vi "Autonomous Independent.vi"() -> ()   [LabVIEW 2015]
doc: "This VI is called when autonomous begins, and will automatically be terminated when autonomous ends. You can carry out timed or sensor driven robot movement independently without needing to return to the caller."
uses:
  <vilib>/Rock Robotics/WPI/Utilities/WPI_GetSetVariantRefNum.vi
  <vilib>/Rock Robotics/Network Tables/NT Write Numeric Array.vi
  <vilib>/Rock Robotics/Network Tables/NT Read Boolean.vi
  <vilib>/Rock Robotics/Network Tables/NT Write Boolean.vi
  <vilib>/Rock Robotics/Network Tables/NT Write Number.vi
  <vilib>/Rock Robotics/Network Tables/NT Read String.vi
  <vilib>/Rock Robotics/WPI/RobotDrive/WPI_RobotDriveArcadeDrive_Standard(NoSaturation).vi
panel:
  out "Current Movement, for debugging":T1 {"Y Joystick Value" scale=1.0..-1.0; "X Joystick Value" scale=-1.0..1.0}
  in  "Array of robot movements":T2(array[cluster])=[{"X Joystick Value"=0.39393939393939403, "Y Joystick Value"=0.0, "Delay (sec)"=1.0, "Movement Name"="turn"}, {"X Joystick Value"=-0.3737373737373737, "Y Joystick Value"=0.0, "Delay (sec)"=1.0, "Movement Name"="turn back"}] {"Y Joystick Value" scale=1.0..-1.0; "X Joystick Value" scale=-1.0..1.0}
  out "Low Switch":bool
  out "High Switch":bool
  out "POT Sensor Meter":dbl(knob) scale=78.0..98.0
  out "POT Sensor Value":dbl
  # "Be sure to right-click and choose Data Operations>>Make Current Value default if you want to save the array values with the VI"
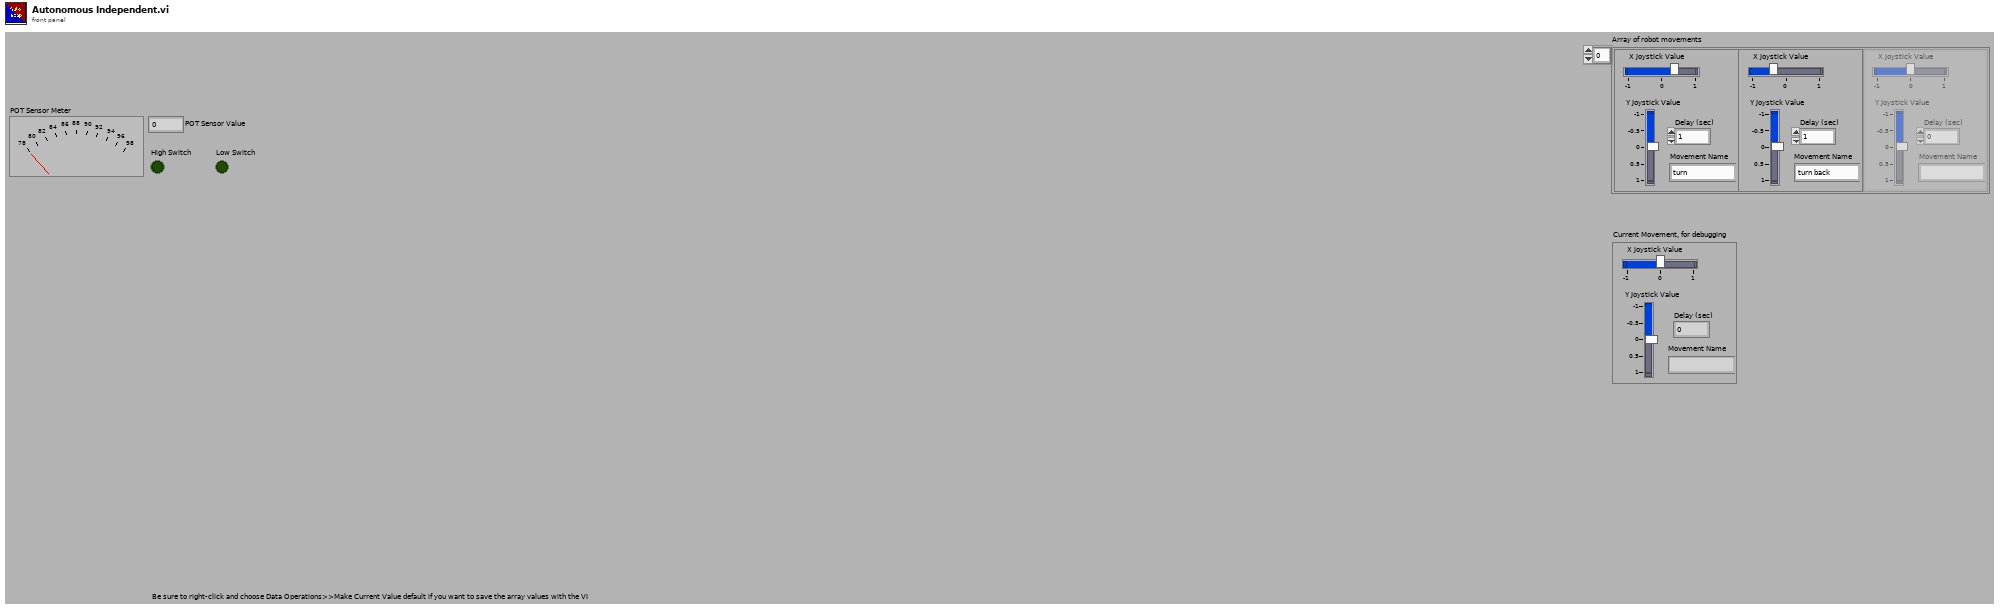
[diagram p1: front panel]
types:
  T1 = cluster{"X Joystick Value":dbl, "Y Joystick Value":dbl, "Delay (sec)":dbl, "Movement Name":string}
  T2 = cluster{"X Joystick Value":dbl, "Y Joystick Value":dbl, "Delay (sec)":dbl, "Movement Name":string}[]
  T3 = typedef "WPI_JoystickDevRef.ctl" = cluster{"Device":T4}
  T4 = typedef "WPI_JoystickDeviceEnum.ctl" = enum16{"USB 0", "USB 1", "USB 2", "USB 3", "USB 4", "USB 5"}
  T5 = typedef "WPI_SwitchDevRef.ctl" = cluster{"DevStatus":errorcluster, "DIO Channel":T6, "CntIndex":T7, "Normally Closed":bool}
  T6 = typedef "FPGA_DIOChannel.ctl" = enum8{"DIO 0", "DIO 1", "DIO 2", "DIO 3", "DIO 4", "DIO 5", "DIO 6", "DIO 7", "DIO 8", "DIO 9", "DIO MXP 0", "DIO MXP 1", "DIO MXP 2", "DIO MXP 3", "DIO MXP 4", "DIO MXP 5", "DIO MXP 6", "DIO MXP 7", "DIO MXP 8", "DIO MXP 9", "DIO MXP 10", "DIO MXP 11", "DIO MXP 12", "DIO MXP 13", "DIO MXP 14", "DIO MXP 15", "Invalid"}
  T7 = typedef "FPGA_CounterCtrSystemIndex.ctl" = enum8{"Ctr 0", "Ctr 1", "Ctr 2", "Ctr 3", "Ctr 4", "Ctr 5", "Ctr 6", "Ctr 7", "Invalid"}
  T8 = typedef "WPI_PotentiometerDevRef.ctl" = cluster{"DevStatus":errorcluster, "Analog Channel":T9, "Invert Output":bool}
  T9 = typedef "FPGA_AIChannel.ctl" = enum8{"AI 0", "AI 1", "AI 2", "AI 3", "AI MXP 0", "AI MXP 1", "AI MXP 2", "AI MXP 3", "Invalid"}
  T10 = typedef "WPI_MotorControlDeviceRef.ctl" = cluster{"DeviceStatus":errorcluster, "Type":T11, "PWM":cluster{"PWM Channel":T12, "DeadBand":T13}, "CAN":cluster{"Device Number":u8, "Control Mode":T14, "Semaphore":T15, "Max Vout":dbl, "TalonSRX Control Mode":T16}, "Invert":bool}
  T11 = typedef "WPI_MotorControlType.ctl" = enum16{"PWM", "CAN", "CANTalonSRX"}
  T12 = typedef "FPGA_DIOPWMChannel.ctl" = enum8{"PWM 0", "PWM 1", "PWM 2", "PWM 3", "PWM 4", "PWM 5", "PWM 6", "PWM 7", "PWM 8", "PWM 9", "PWM MXP 0", "PWM MXP 1", "PWM MXP 2", "PWM MXP 3", "PWM MXP 4", "PWM MXP 5", "PWM MXP 6", "PWM MXP 7", "PWM MXP 8", "PWM MXP 9", "Invalid"}
  T13 = typedef "WPI_PWMDeadband.ctl" = cluster{"Name":string, "maxPositivePwm":i32, "minPositivePwm":i32, "centerPwm":i32, "maxNegativePwm":i32, "minNegativePwm":i32, "angularRange":u16}
  T14 = typedef "WPI_CANJaguar_ControlMode.ctl" = enum8{"Percent VBus", "Current", "Speed", "Position", "Voltage"}
  T15 = typedef "Semaphore RefNum" = refnum<k1>
  T16 = typedef "WPI_CANTalonSRX_APIControlMode.ctl" = enum8{"Percent VBus", "Speed", "Position", "Slave", "Unchanged / Invalid", "Voltage Compensation", "Current", "Motion Profile"}
  T17 = typedef "WPI_RobotDriveDevRef.ctl" = cluster{"DevStatus":errorcluster, "Motors[]":T10[], "Square Inputs":bool, "Max Output":dbl}
  T18 = typedef "WPI_CounterDevRef.ctl" = cluster{"DevStatus":errorcluster, "CntIndex":T7}
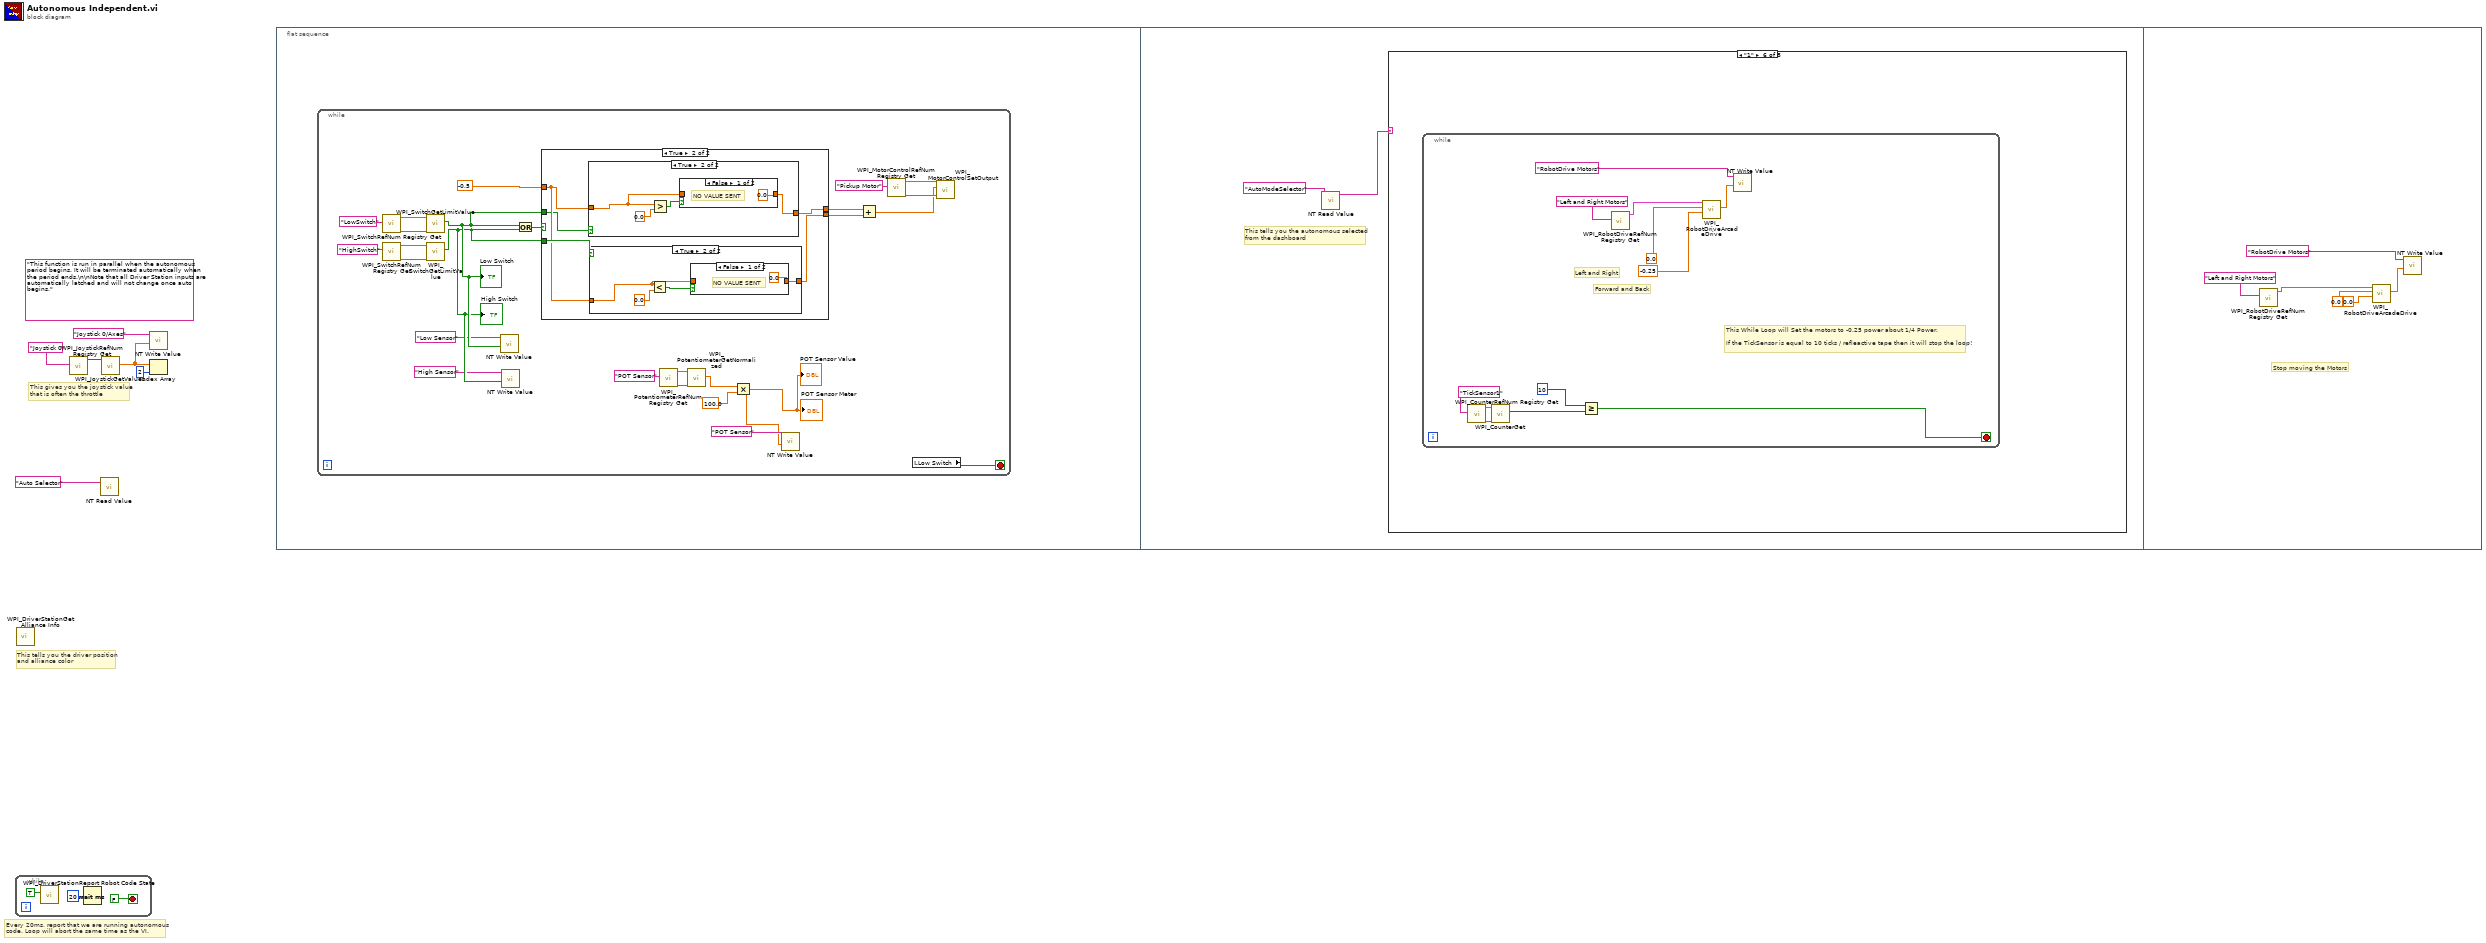
[diagram p0: block diagram]
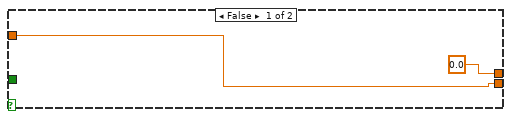
[diagram p2: hidden frame]
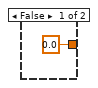
[diagram p3: hidden frame]
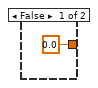
[diagram p5: hidden frame]
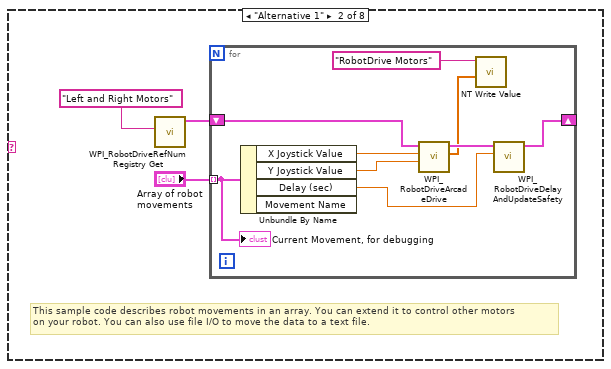
[diagram p8: hidden frame]
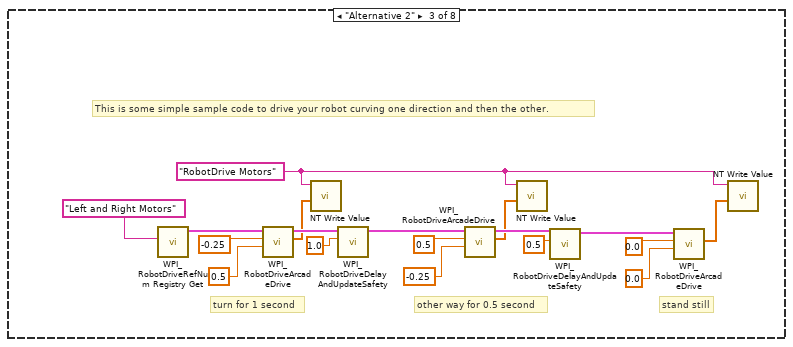
[diagram p9: hidden frame]
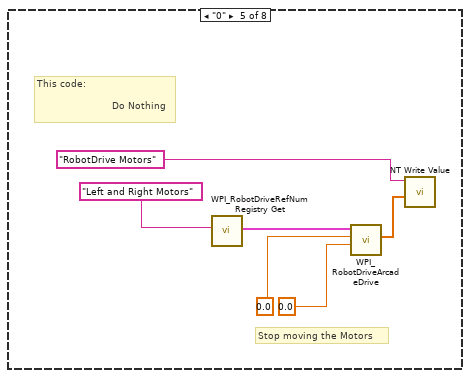
[diagram p11: hidden frame]
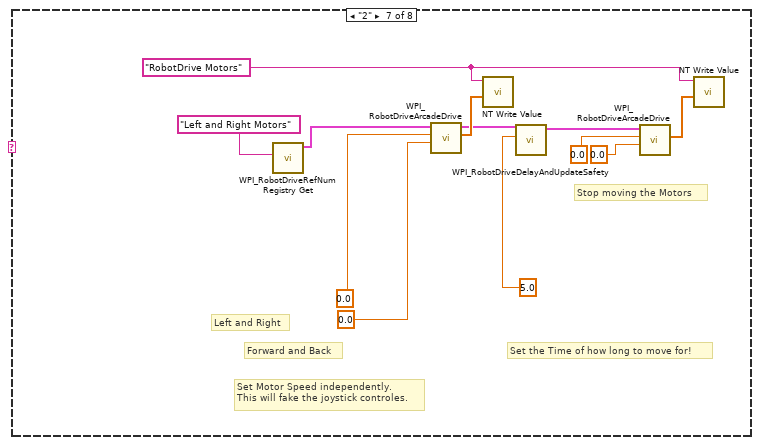
[diagram p12: hidden frame]
diagram:
  (unwired) "This function is run in parallel when the autonomous period begins. It will be terminated automatically when the period ends.\n\nNote that all Driver Station inputs are automatically latched and will not change once auto begins."
  # "Every 20ms, report that we are running autonomous\ncode. Loop will abort the same time as the VI."
  # "This gives you the joystick value\nthat is often the throttle"
  # "This tells you the driver position\nand alliance color"
  n1 = while {
    stop <- FALSE stop-if-true
    n2 = call <vilib>:"WPI_DriverStationReport Robot Code State.vi"("Autonomous"=TRUE) -> ()  [unwired: 10 in, 1 out]
    n3 = Wait (ms)(milliseconds to wait=u32 20) -> ()  [unwired: 1 out]
  }
  n4 = call <vilib>:"WPI_DriverStationGet Alliance Info.vi"() -> ()  [unwired: 12 out]
  n5 = call <vilib>:"WPI_JoystickRefNum Registry Get.vi"("refnum name"="Joystick 0") -> ("JoystickDevRef"=w5:T3)  [unwired: 1 in, 9 out]
  n6 = call-poly <vilib>:"NT Read Value.vi"("Name"="Auto Selector") -> ()  [unwired: 9 in, 2 out]
  n7 = call <vilib>:"WPI_JoystickGetValues.vi"("JoystickDevRef"=w5) -> ("Axes"=w3:dbl[])  [unwired: 6 in, 4 out]
  n8 = call-poly <vilib>:"NT Write Value.vi"("Numeric Array"=w3, "Name"="Joystick 0/Axes") -> ()  [unwired: 9 in, 1 out]
  n9 = Index Array(array=w3, index=2) -> ()  [unwired: 1 out]
  n10 = flat-sequence {
    frame #0 {
      n11 = while {
        stop <- w10 stop-if-true
        n12 = call <vilib>:"WPI_SwitchRefNum Registry Get.vi"("refnum name"="LowSwitch") -> ("error out"=w33:errorcluster, "SwitchDevRef"=w34:T5)  [unwired: 9 in]
        n13 = call <vilib>:"WPI_SwitchRefNum Registry Get.vi"("refnum name"="HighSwitch") -> ("error out"=w30:errorcluster, "SwitchDevRef"=w31:T5)  [unwired: 9 in]
        n14 = call <vilib>:"WPI_SwitchGetLimitValue.vi"("error in (no error)"=w33, "SwitchDevRef"=w34) -> ("Switch Pressed"=w18:bool)  [unwired: 7 in, 2 out]
        "Low Switch" <- w18
        n15 = call <vilib>:"WPI_SwitchGetLimitValue.vi"("error in (no error)"=w30, "SwitchDevRef"=w31) -> ("Switch Pressed"=w17:bool)  [unwired: 7 in, 2 out]
        "High Switch" <- w17
        n16 = call-poly <vilib>:"NT Write Value.vi"("Boolean"=w18, "Name"="Low Sensor") -> ()  [unwired: 9 in, 1 out]
        n17 = call-poly <vilib>:"NT Write Value.vi"("Boolean"=w17, "Name"="High Sensor") -> ()  [unwired: 9 in, 1 out]
        n18 = Or(x=w18, y=w17) -> (x .or. y?=w35:bool)
        n19 = case shown="True" w35 {
          tunnel: w18 -> [_ w40]
          tunnel: w17 -> [_ w42]
          tunnel: -0.5 ("Axes[1]") -> [w36 w41]
          tunnel: [0.0 ("Axes[1]") w39] -> w24
          tunnel: [w36 w38] -> w23
          frame False {
          }
          frame True {
            n20 = case shown="True" w40 {
              tunnel: w41 -> [_ w52]
              tunnel: [0.0 ("Axes[1]") w51] -> w39
              frame False {
              }
              frame True {
                n21 = Greater?(x=w52, y=0.0) -> (0:w53:bool)
                n22 = case shown="False" w53 {
                  tunnel: [0.0 ("Axes[1]") w56] -> w51
                  tunnel: w52 -> [_ w56]
                  frame False {
                    # "NO VALUE SENT"
                  }
                  frame True {
                  }
                }
              }
            }
            n23 = case shown="True" w42 {
              tunnel: w41 -> [_ w44]
              tunnel: [0.0 ("Axes[1]") w45] -> w38
              frame False {
              }
              frame True {
                n24 = Less?(x=w44, y=0.0) -> (x < y?=w46:bool)
                n25 = case shown="False" w46 {
                  tunnel: [0.0 ("Axes[1]") w49] -> w45
                  tunnel: w44 -> [_ w49]
                  frame False {
                    # "NO VALUE SENT"
                  }
                  frame True {
                  }
                }
              }
            }
          }
        }
        n26 = call <vilib>:"WPI_PotentiometerRefNum Registry Get.vi"("refnum name"="POT Sensor") -> ("error out"=w22:errorcluster, "PotDevRef"=w21:T8)  [unwired: 9 in]
        n27 = call <vilib>:"WPI_PotentiometerGetNormalized.vi"("error in"=w22, "PotDevRef"=w21) -> ("Normalized Value"=w14:dbl)  [unwired: 7 in, 2 out]
        n28 = Multiply(x=w14, y=100.0) -> (x*y=w12:dbl)
        "POT Sensor Value" <- w12
        "POT Sensor Meter" <- w12
        n29 = call-poly <vilib>:"NT Write Value.vi"("Numeric"=w12, "Name"="POT Sensor") -> ()  [unwired: 9 in, 1 out]
        n30 = Add(x=w24, y=w23) -> (x+y=w25:dbl)
        n31 = call <vilib>:"WPI_MotorControlRefNum Registry Get.vi"("refnum name"="Pickup Motor") -> ("error out"=w28:errorcluster, "MotorControlDevRef"=w27:T10)  [unwired: 9 in]
        n32 = local read "Low Switch"() -> (w10:bool)
        n33 = call <vilib>:"WPI_MotorControlSetOutput.vi"("error in (no error)"=w28, "Output"=w25, "MotorControlDevRef"=w27) -> ()  [unwired: 6 in, 3 out]
      }
    }
    frame #1 {
      # "This tells you the autonomous selected\nfrom the dashboard"
      n34 = call-poly <vilib>:"NT Read Value.vi"("Name"="AutoModeSelector") -> ("String"=w57:string)  [unwired: 9 in, 1 out]
      n35 = case shown="\"1\"" w57 {
        frame Default {
          # "You can put your main auto here, or you can right-click on the case and make any\nother frame be the default case."
          # "This is the frame that will execute if no selection is made, or if it is not recognized"
        }
        frame "Alternative 1" {
          # "This sample code describes robot movements in an array. You can extend it to control other motors\non your robot. You can also use file I/O to move the data to a text file."
          n36 = call <vilib>:"WPI_RobotDriveRefNum Registry Get.vi"("refnum name"="Left and Right Motors") -> ("RobotDriveDevRef"=w60:T17)  [unwired: 1 in, 9 out]
          n37 = for {
            shift-right: [w68] -> _
            shift-left: w60 -> [w69]
            tunnel: "Array of robot movements" -> [w64] mode=indexing
            n38 = Unbundle By Name(w64) -> ("X Joystick Value"=w67:dbl, "Y Joystick Value"=w66:dbl, "Delay (sec)"=w65:dbl)  [unwired: 1 out]
            n39 = call-poly <vilib>:"WPI_RobotDriveArcadeDrive.vi"("Y axis value"=w66, "X axis value"=w67, "RobotDriveDevRef"=w69) -> ("Motor Values"=w62:dbl[], "RobotDriveDevRef"=w70:T17)  [unwired: 1 in, 6 out]
            n40 = call-poly <vilib>:"NT Write Value.vi"("Numeric Array"=w62, "Name"="RobotDrive Motors") -> ()  [unwired: 9 in, 1 out]
            n41 = call <vilib>:"WPI_RobotDriveDelayAndUpdateSafety.vi"("Delay (s)"=w65, "RobotDriveDevRef"=w70) -> ("RobotDriveDevRef 2"=w68:T17)  [unwired: 8 in, 1 out]
            "Current Movement, for debugging" <- w64
          }
        }
        frame "Alternative 2" {
          w72 = "RobotDrive Motors" ("Name")
          # "This is some simple sample code to drive your robot curving one direction and then the other."
          # "stand still"
          # "other way for 0.5 second"
          # "turn for 1 second"
          n42 = call <vilib>:"WPI_RobotDriveRefNum Registry Get.vi"("refnum name"="Left and Right Motors") -> ("RobotDriveDevRef"=w88:T17)  [unwired: 1 in, 9 out]
          n43 = call-poly <vilib>:"WPI_RobotDriveArcadeDrive.vi"("Y axis value"=0.5 ("X axis value"), "X axis value"=-0.25, "RobotDriveDevRef"=w88) -> ("Motor Values"=w71:dbl[], "RobotDriveDevRef"=w81:T17)  [unwired: 1 in, 6 out]
          n44 = call-poly <vilib>:"NT Write Value.vi"("Numeric Array"=w71, "Name"=w72) -> ()  [unwired: 9 in, 1 out]
          n45 = call <vilib>:"WPI_RobotDriveDelayAndUpdateSafety.vi"("Delay (s)"=1.0, "RobotDriveDevRef"=w81) -> ("RobotDriveDevRef 2"=w82:T17)  [unwired: 8 in, 1 out]
          n46 = call-poly <vilib>:"WPI_RobotDriveArcadeDrive.vi"("Y axis value"=-0.25 ("X axis value"), "X axis value"=0.5, "RobotDriveDevRef"=w82) -> ("Motor Values"=w73:dbl[], "RobotDriveDevRef"=w83:T17)  [unwired: 1 in, 6 out]
          n47 = call-poly <vilib>:"NT Write Value.vi"("Numeric Array"=w73, "Name"=w72) -> ()  [unwired: 9 in, 1 out]
          n48 = call <vilib>:"WPI_RobotDriveDelayAndUpdateSafety.vi"("Delay (s)"=0.5, "RobotDriveDevRef"=w83) -> ("RobotDriveDevRef 2"=w84:T17)  [unwired: 8 in, 1 out]
          n49 = call-poly <vilib>:"WPI_RobotDriveArcadeDrive.vi"("Y axis value"=0.0 ("X axis value"), "X axis value"=0.0, "RobotDriveDevRef"=w84) -> ("Motor Values"=w74:dbl[])  [unwired: 1 in, 7 out]
          n50 = call-poly <vilib>:"NT Write Value.vi"("Numeric Array"=w74, "Name"=w72) -> ()  [unwired: 9 in, 1 out]
        }
        frame "Your Turn" {
        }
        frame "0" {
          # "Stop moving the Motors"
          # "This code:\n                   \n                         Do Nothing"
          n51 = call <vilib>:"WPI_RobotDriveRefNum Registry Get.vi"("refnum name"="Left and Right Motors") -> ("RobotDriveDevRef"=w89:T17)  [unwired: 1 in, 9 out]
          n52 = call-poly <vilib>:"WPI_RobotDriveArcadeDrive.vi"("Y axis value"=0.0 ("X axis value"), "X axis value"=0.0, "RobotDriveDevRef"=w89) -> ("Motor Values"=w93:dbl[])  [unwired: 1 in, 7 out]
          n53 = call-poly <vilib>:"NT Write Value.vi"("Numeric Array"=w93, "Name"="RobotDrive Motors") -> ()  [unwired: 9 in, 1 out]
        }
        frame "1" {
          n54 = while {
            stop <- w101 stop-if-true
            # "This While Loop will Set the motors to -0.25 power about 1/4 Power.\n\nIf the TickSensor is equal to 10 ticks / refleactive tape then it will stop the loop!"
            # "Forward and Back"
            # "Left and Right"
            n55 = call <vilib>:"WPI_CounterRefNum Registry Get.vi"("refnum name"="TickSensor1") -> ("error out"=w105:errorcluster, "CounterDevRef"=w104:T18)  [unwired: 9 in]
            n56 = call <vilib>:"WPI_CounterGet.vi"("error in (no error)"=w105, "CounterDevRef in"=w104) -> ("Value"=w103:i32)  [unwired: 4 in, 5 out]
            n57 = Greater Or Equal?(x=10, y=w103) -> (x >= y?=w101:bool)
            n58 = call <vilib>:"WPI_RobotDriveRefNum Registry Get.vi"("refnum name"="Left and Right Motors") -> ("RobotDriveDevRef"=w100:T17)  [unwired: 1 in, 9 out]
            n59 = call-poly <vilib>:"WPI_RobotDriveArcadeDrive.vi"("Y axis value"=-0.25 ("X axis value"), "X axis value"=0.0, "RobotDriveDevRef"=w100) -> ("Motor Values"=w98:dbl[])  [unwired: 1 in, 7 out]
            n60 = call-poly <vilib>:"NT Write Value.vi"("Numeric Array"=w98, "Name"="RobotDrive Motors") -> ()  [unwired: 9 in, 1 out]
          }
        }
        frame "2" {
          w117 = "RobotDrive Motors" ("Name")
          # "Forward and Back"
          # "Left and Right"
          # "Set Motor Speed independently.\nThis will fake the joystick controles."
          # "Set the Time of how long to move for!"
          # "Stop moving the Motors"
          n61 = call <vilib>:"WPI_RobotDriveRefNum Registry Get.vi"("refnum name"="Left and Right Motors") -> ("RobotDriveDevRef"=w118:T17)  [unwired: 1 in, 9 out]
          n62 = call-poly <vilib>:"WPI_RobotDriveArcadeDrive.vi"("Y axis value"=0.0 ("X axis value"), "X axis value"=0.0, "RobotDriveDevRef"=w118) -> ("Motor Values"=w116:dbl[], "RobotDriveDevRef"=w110:T17)  [unwired: 1 in, 6 out]
          n63 = call-poly <vilib>:"NT Write Value.vi"("Numeric Array"=w116, "Name"=w117) -> ()  [unwired: 9 in, 1 out]
          n64 = call <vilib>:"WPI_RobotDriveDelayAndUpdateSafety.vi"("Delay (s)"=5.0, "RobotDriveDevRef"=w110) -> ("RobotDriveDevRef 2"=w109:T17)  [unwired: 8 in, 1 out]
          n65 = call-poly <vilib>:"WPI_RobotDriveArcadeDrive.vi"("Y axis value"=0.0 ("X axis value"), "X axis value"=0.0, "RobotDriveDevRef"=w109) -> ("Motor Values"=w115:dbl[])  [unwired: 1 in, 7 out]
          n66 = call-poly <vilib>:"NT Write Value.vi"("Numeric Array"=w115, "Name"=w117) -> ()  [unwired: 9 in, 1 out]
        }
        frame "3" {
        }
      }
    }
    frame #2 {
      # "Stop moving the Motors"
      n67 = call <vilib>:"WPI_RobotDriveRefNum Registry Get.vi"("refnum name"="Left and Right Motors") -> ("RobotDriveDevRef"=w119:T17)  [unwired: 1 in, 9 out]
      n68 = call-poly <vilib>:"WPI_RobotDriveArcadeDrive.vi"("Y axis value"=0.0 ("X axis value"), "X axis value"=0.0, "RobotDriveDevRef"=w119) -> ("Motor Values"=w121:dbl[])  [unwired: 1 in, 7 out]
      n69 = call-poly <vilib>:"NT Write Value.vi"("Numeric Array"=w121, "Name"="RobotDrive Motors") -> ()  [unwired: 9 in, 1 out]
    }
  }
